vi "[GV]_GPS Raw_Lon.vi"() -> ()   [LabVIEW 2016]
panel:
  out "GPS Raw_Lon":dbl format="%.8f"
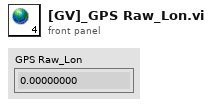
[diagram p1: front panel]
diagram:
